vi "setNewTemperature.vi"(8 "error in (no error)":errorcluster, 9 "releaseWhenReady":bool, 10 "temperature":dbl, 11 "CameraManager in":refnum<class "CameraManager.lvclass">) -> (0 "error out":errorcluster, 3 "CameraManager out":refnum<class "CameraManager.lvclass">)   [LabVIEW 2009, in "iManagement.lvlib" / "CameraManager.lvclass"]
uses:
  CameraManager.lvclass
  CameraManager.lvclass/CameraManager.ctl
  Hal/Channels/Camera/CameraController.lvclass
  Hal/Channels/Camera/CameraEventsManager/CameraEventsManger.lvclass
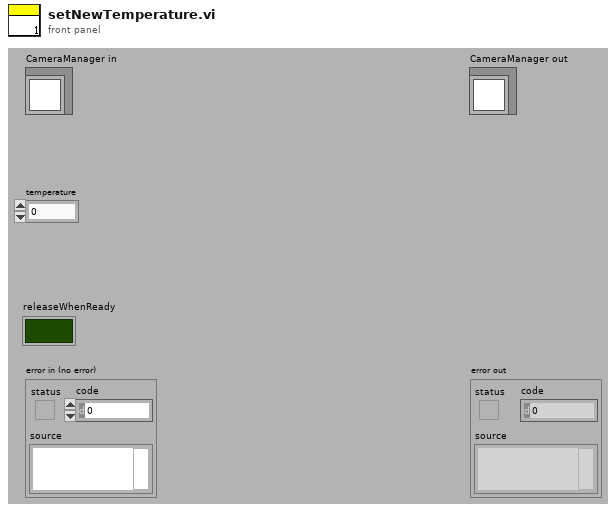
[diagram p1: front panel]
types:
  T1 = cluster{"newSetPointEvent":refnum<user-event>, "stopCoolingEvent":refnum<user-event>}
  T2 = cluster{"closeEvent":refnum<user-event>, "temperatureUpdateEvent":refnum<user-event>, "displayErrorEvent":refnum<user-event>, "setPointUpdateEvent":refnum<user-event>}
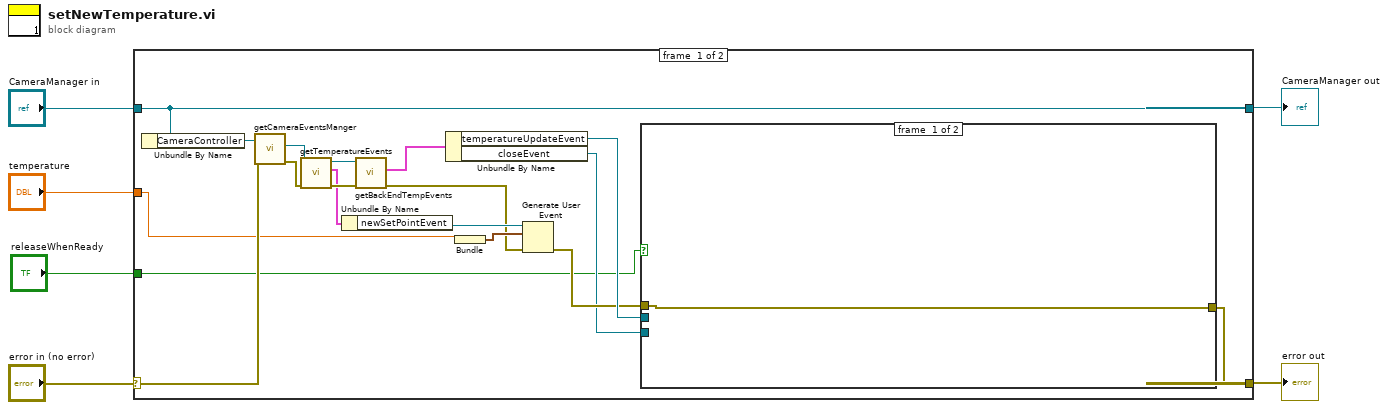
[diagram p0: block diagram]
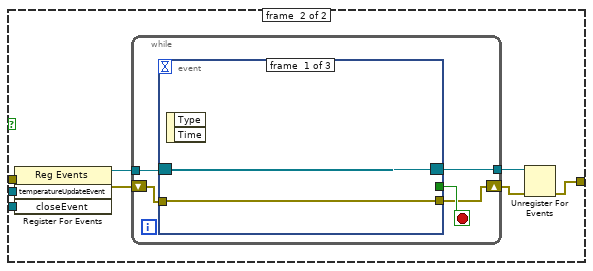
[diagram p2: hidden frame]
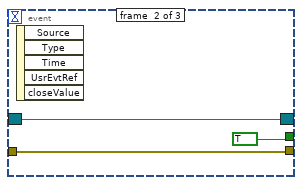
[diagram p3: hidden frame]
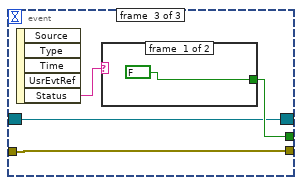
[diagram p4: hidden frame]
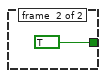
[diagram p5: hidden frame]
diagram:
  n1 = case shown="No Error" "error in (no error)" {
    selector: "error in (no error)" -> [w22 w51]
    tunnel: [w8 w51] -> w5
    tunnel: [w24 w50] -> w3
    tunnel: "CameraManager in" -> [w24 w50]
    tunnel: "temperature" -> [w16 _]
    tunnel: "releaseWhenReady" -> [w9 _]
    frame #0 {
      n2 = Unbundle By Name(w24) -> ("CameraController"=w23:refnum<class "CameraController.lvclass">)
      n3 = call-dynamic "getCameraEventsManger.vi"("error in (no error)"=w22, "CameraController.lvclass in"=w23) -> ("error out"=w14:errorcluster, "Hardware:Channels.lvlib:CameraEventsManger.lvclass"=w21:refnum<class "CameraEventsManger.lvclass">)  [unwired: 7 in, 1 out]
      n4 = call-dynamic "getTemperatureEvents.vi"("error in (no error)"=w14, "CameraEventsManger.lvclass in"=w21) -> ("error out"=w20:errorcluster, "temperatureEvents"=w7:T1, "CameraEventsManger.lvclass out"=w19:refnum<class "CameraEventsManger.lvclass">)  [unwired: 7 in]
      n5 = Unbundle By Name(w7) -> ("newSetPointEvent"=w18:refnum<user-event>)
      n6 = call-dynamic "getBackEndTempEvents.vi"("error in (no error)"=w20, "CameraEventsManger.lvclass in"=w19) -> ("error out"=w15:errorcluster, "backEndTempEvents"=w13:T2)  [unwired: 7 in, 1 out]
      n7 = Unbundle By Name(w13) -> ("temperatureUpdateEvent"=w12:refnum<user-event>, "closeEvent"=w10:refnum<user-event>)
      n8 = Bundle("temperature"=w16) -> (w17:cluster{"temperature":dbl})  [unwired: 1 in]
      n9 = Generate User Event(user event=w18, event data cluster=w17, error in=w15) -> (error out=w11:errorcluster)  [unwired: 1 out]
      n10 = case shown="True" w9 {
        tunnel: w12 -> [_ w33]
        tunnel: w11 -> [w25 w32]
        tunnel: w10 -> [_ w29]
        tunnel: [w25 w26] -> w8
        frame #0 {
        }
        frame #1 {
          n11 = register-events(error in=w32, w33, w29) -> (reference out=w31:refnum<event-registration>, error out=w30:errorcluster)  [unwired: 1 in]
          n12 = while {
            tunnel: w31 -> [w38]
            shift-right: [w35] -> w27
            shift-left: w30 -> [w37]
            tunnel: [w34] -> w28
            stop <- w36 stop-if-true
            n13 = event shown="[2] <temperatureUpdateEvent>: User Event" {
              selector: w38 -> [w40 w43 w45]
              dyn-events: [w40 w43 w45] -> w34
              timeout: _ -> [_ _ _]
              tunnel: w37 -> [w39 w41 w44]
              tunnel: [_ TRUE w46] -> w36
              tunnel: [w39 w41 w44] -> w35
              event #0 {
                n14 = event-data() -> ()  [unwired: 1 in, 2 out]
              }
              event #1 {
                n15 = event-data() -> ()  [unwired: 1 in, 5 out]
              }
              event #2 {
                n16 = event-data() -> ("Status"=w47:string)  [unwired: 1 in, 4 out]
                n17 = case shown="\"TEMP_STABILIZED\"" w47 {
                  tunnel: [FALSE TRUE] -> w46
                  frame #0 {
                  }
                  frame #1 {
                  }
                }
              }
            }
          }
          n18 = Unregister For Events(event registration refnum=w28, error in=w27) -> (error out=w26:errorcluster)
        }
      }
    }
    frame #1 {
    }
  }
  "error out" <- w5
  "CameraManager out" <- w3
